vi "new Dashboard Main.vi"() -> ()   [LabVIEW 2020]
uses:
  <vilib>/Rock Robotics/Network Tables/NT Read Numeric Array.vi
panel:
  out "Camera Perf":string
  in  "Camera Settings":T1={"Frame Rate"=30, "Compression"=30, "Size"=1, "DB Camera Config"=FALSE} {"Frame Rate" scale=1.0..30.0; "Compression" scale=100.0..-1.0; "Size" items=["640x480", "320x240", "160x120"]}
  in  "TCP":refnum<k5>
  out "Robot IP":string
  in  "Dashboard Tab":enum32{"Drive", "Basic", "Custom", "Variables"}(tab)
  in  "Select Auto":string(combo)="Select Autonomous ..."
  out "NT Connection":bool
  out "MotorChart R":cluster{"Numeric":dbl, "Numeric":dbl}(graph)
  out "MotorChart L":cluster{"Numeric":dbl, "Numeric":dbl}(graph)
  out "MotorSliders R":cluster{"MotorSlide1":dbl, "MotorSlide2":dbl} {"MotorSlide2" scale=-1.0..1.0 scale format="%#_2e"; "MotorSlide1" scale=-1.0..1.0 scale format="%#_2e"}
  out "MotorSliders L":cluster{"MotorSlide1":dbl, "MotorSlide2":dbl} {"MotorSlide2" scale=-1.0..1.0 scale format="%#_2e"; "MotorSlide1" scale=-1.0..1.0 scale format="%#_2e"}
  out "JS1 Z":dbl(slide) scale=-1.0..1.0 scale format="%#_2e"
  out "JS1 Graph":cluster{"X":dbl, "Y":dbl}[](graph)
  out "JS1 Buttons":T2
  out "JS2 Z":dbl(slide) scale=-1.0..1.0 scale format="%#_2e"
  out "JS2 Graph":cluster{"X":dbl, "Y":dbl}[](graph)
  out "JS2 Buttons":T2
  out "Mode":T3(ring)=enum."Auto Disabled"
  in  "DB/String 9":string
  in  "DB/String 8":string
  in  "DB/String 7":string
  in  "DB/String 6":string
  in  "DB/String 5":string
  in  "DB/String 4":string
  in  "DB/String 3":string
  in  "DB/String 2":string
  in  "DB/String 1":string
  in  "DB/String 0":string
  in  "DB/Slider 0":dbl(slide) scale=0.0..5.0
  in  "DB/Slider 1":dbl(slide) scale=0.0..5.0
  in  "DB/Slider 2":dbl(slide) scale=0.0..5.0
  in  "DB/Slider 3":dbl(slide) scale=0.0..5.0
  out "DB/LED 3":bool
  out "DB/LED 2":bool
  out "DB/LED 1":bool
  out "DB/LED 0":bool
  in  "DB/Button 3":bool
  in  "DB/Button 2":bool
  in  "DB/Button 1":bool
  in  "DB/Button 0":bool
  out "Tree":string(tree)
  out "Camera Image":T4(plugin-control)
  out "Background":bool
  in  "Camera Name":string(combo)="No Camera Selection"
  # "HW"
  # "Joysticks"
  # "Drive Motors"
  # "Front"
  # "Right"
  # "Left"
  # "Back"
  # "This tab is a great place for autonomous settings and robot-specific values.\nPlace controls and indicators inside this tab and match name to\nDashboard Variables on robot. You can also delete this comment."
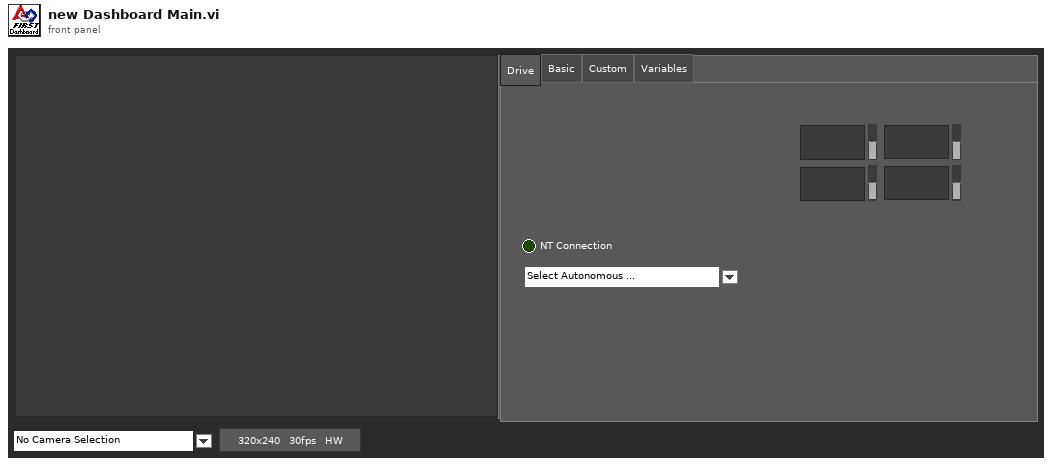
[diagram p1: front panel]
types:
  T1 = cluster{"Frame Rate":i32, "Compression":i32, "Size":u16, "DB Camera Config":bool}
  T2 = cluster{bool, bool, bool, bool, bool, bool, bool, bool, bool, bool, bool, bool}
  T3 = enum8{"Tele-Op Disabled", "Tele-Op Enabled", "Auto Disabled", "Auto Enabled", "Test Disabled", "Test Enabled", "Disconnected", "No Code", "E-Stop"}
  T4 = typedef "IMAQ Image.ctl" = refnum<image>
  T5 = cluster{"Save Path":path, "Interval (s)":dbl, "Keep":i32}
  T6 = typedef "Image Type" = u32
  T7 = cluster{"Camera Image":refnum<vi>, "Dashboard Tab":refnum<vi>, "Background":refnum<vi>, "Tree":refnum<vi>, "Camera Settings":refnum<vi>, "Camera Name":refnum<vi>, "Camera Perf":refnum<vi>}
  T8 = cluster{"Shift":bool, "Ctrl":bool, "Alt":bool, "Cmd":bool, "Opt":bool}
  T9 = cluster{"Error Strings":string, "Disable Counts":cluster{u16, u16}, "Rail Faults":cluster{u16, u16, u16}, "Robot IP":string, "DB Mode":u8, "Event Info":cluster{"Name":string, "Type":u8, "Number":u16, "Replay":u8}}
  T10 = cluster{"Storage":cluster{"Disk Free":u64, "RAM Block":u32, "RAM free":u32}, "CPU Utilization":cluster{"CPU % ISR":sgl, "CPU % Time Crit":sgl, "CPU % Timed Str":sgl, "CPU % High":sgl, "CPU % Above":sgl, "CPU % Normal":sgl, "CPU % Low":sgl}, "CAN":cluster{"% Bus Utilization":sgl, "Bus Off Cnt":u32, "TX_FIFO Full Cnt":u32, "Receive Error Cnt":u8, "Transmit Error Cnt":u8}, "HID":cluster{"HID Outputs":u32, "Rumble Low":u16, "Rumble High":u16}[]}
  T11 = cluster{"Status bits":cluster{"Test Mode":bool, "Autonomous":bool, "Enabled":bool, "Code Start":bool, "Brownout":bool, "Reserved 2":bool, "Reserved 3":bool, "E-Stop":bool}, "Code Trace":cluster{"Disabled":bool, "TeleOp":bool, "Auto":bool, "Test":bool}, "Controller Type":enum16{"unknown", "cRIO", "roboRio"}, "Code?":enum16{"unknown", "noCode", "code"}, "Battery V":dbl}
  T12 = cluster{"Control Bits":cluster{"TestMode":bool, "Autonomous":bool, "Enabled":bool, "FMS Present":bool, bool, bool, bool, "E-Stop":bool}, "Team Station ":u8, "Countdown":sgl, "Joystick Values":cluster{"Axes":dbl[], "Buttons":bool[], "POVs":i16[]}[]}
  T13 = cluster{"Axes":dbl[], "Buttons":bool[], "POVs":i16[]}[]
  T14 = cluster{"Axes":dbl[], "Buttons":bool[], "POVs":i16[]}
  T15 = cluster{"Buttons[0]":bool, "Buttons[1]":bool, "Buttons[2]":bool, "Buttons[3]":bool, "Buttons[4]":bool, "Buttons[5]":bool, "Buttons[6]":bool, "Buttons[7]":bool, "Buttons[8]":bool, "Buttons[9]":bool, "Buttons[10]":bool, "Buttons[11]":bool}
  T16 = cluster{"Camera Name":string, "Camera File Name":string, "Saved DB Images Info":cluster{"Save Path":path, "Interval (s)":dbl, "Keep":i32}}
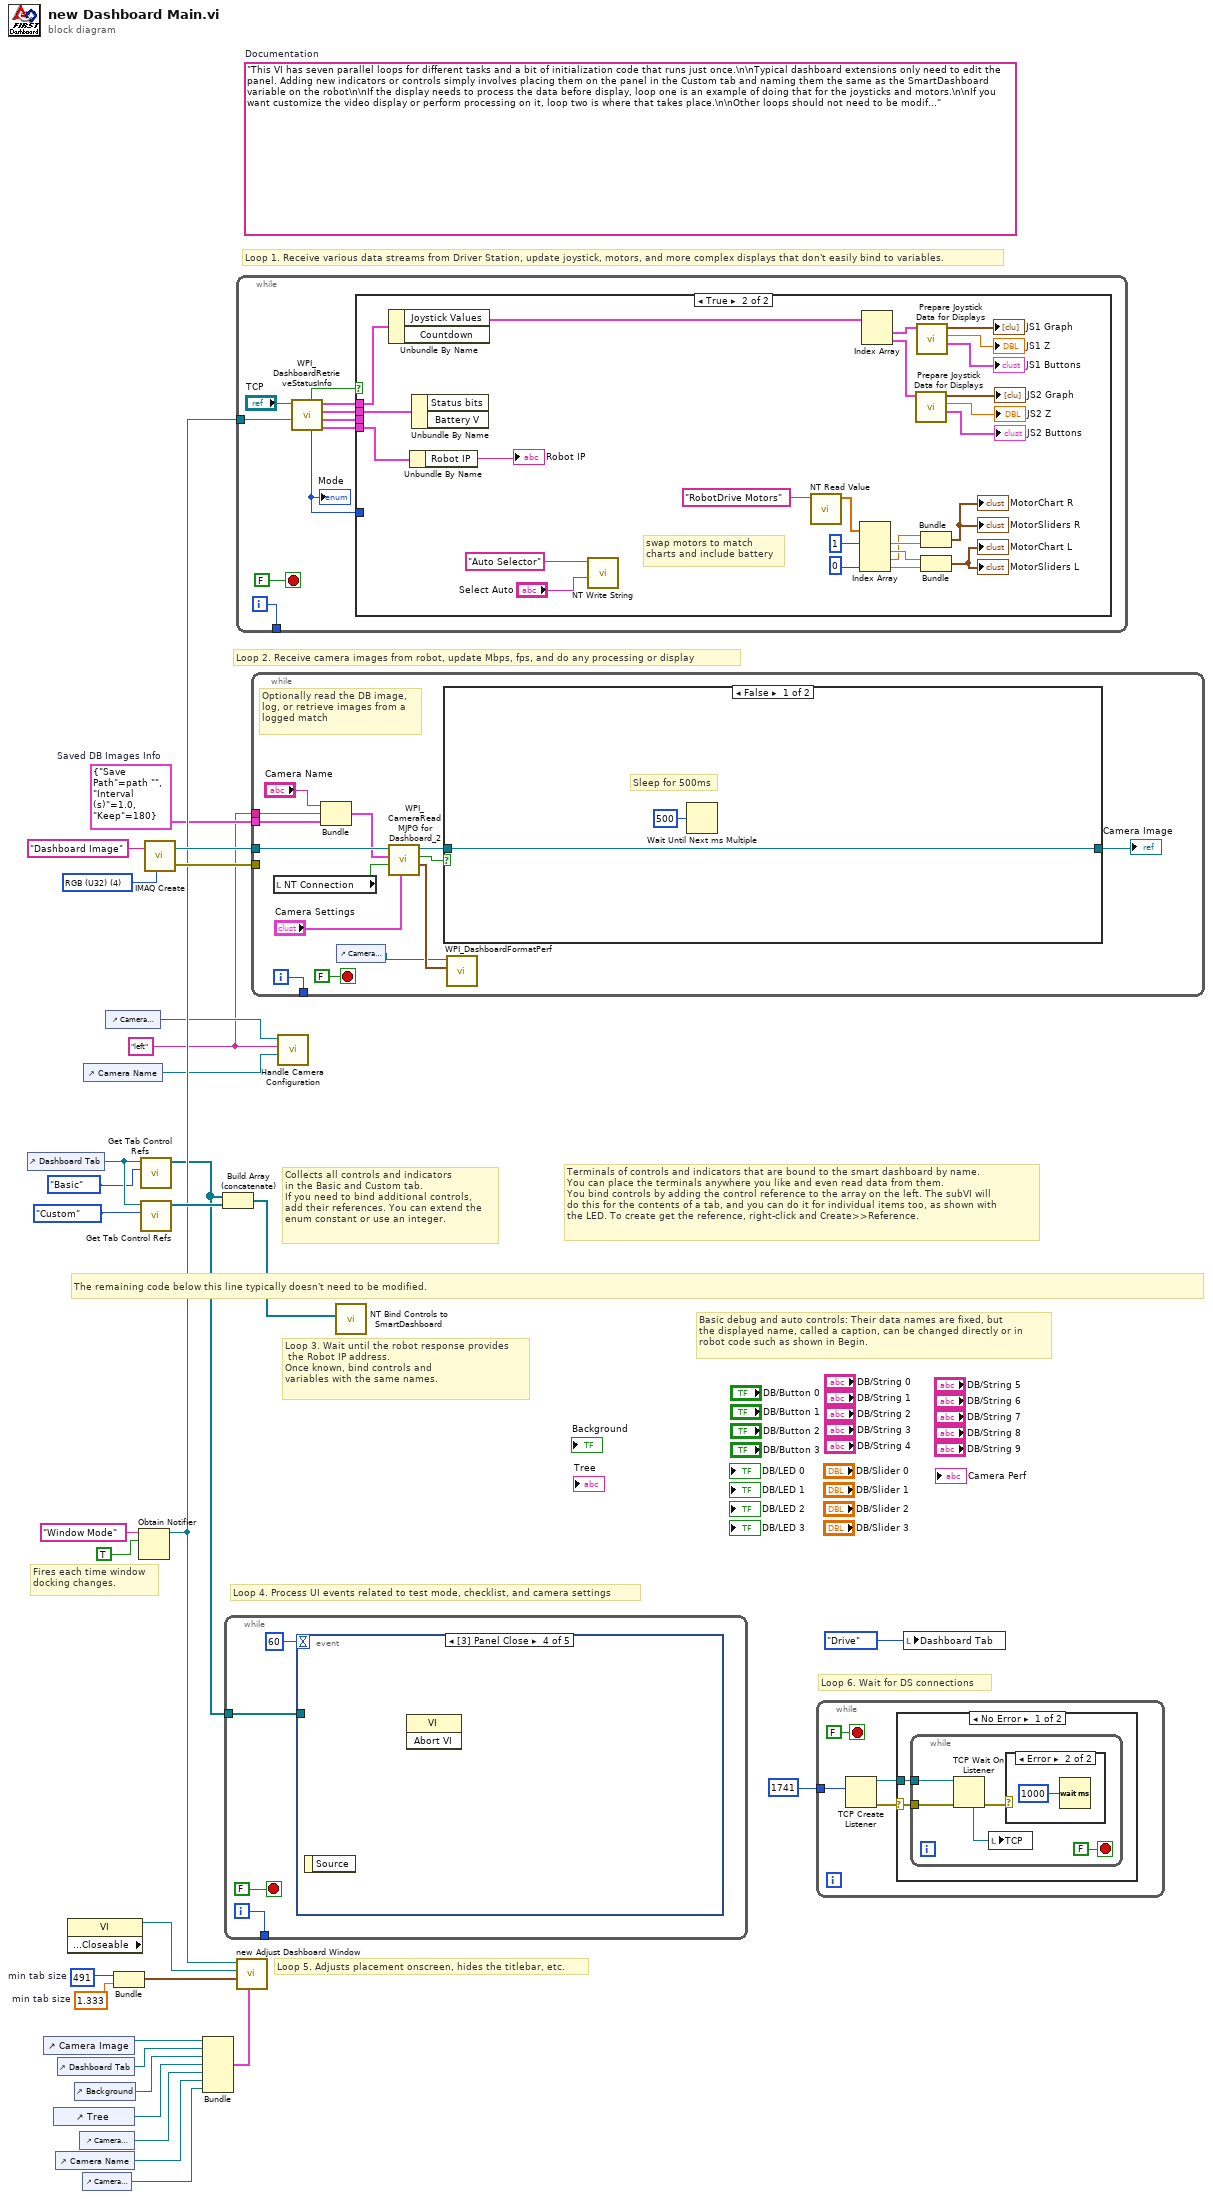
[diagram p0: block diagram]
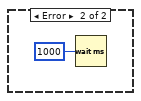
[diagram p3: hidden frame]
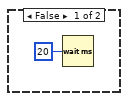
[diagram p4: hidden frame]
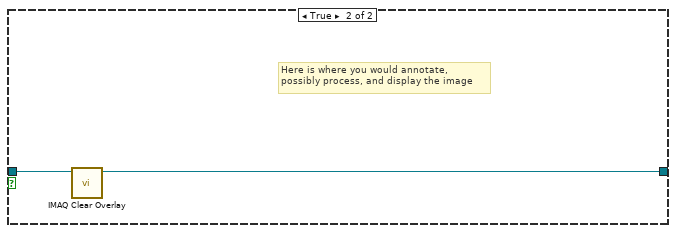
[diagram p5: hidden frame]
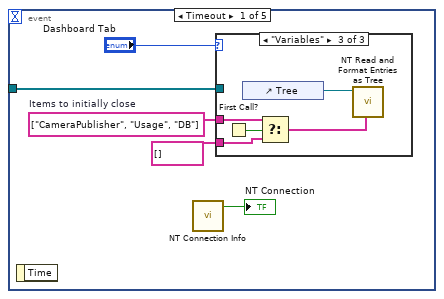
[diagram p6: hidden frame]
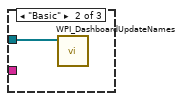
[diagram p8: hidden frame]
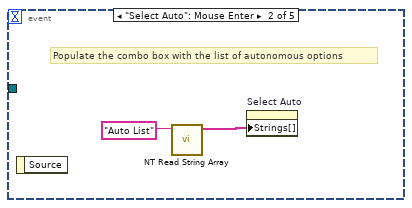
[diagram p9: hidden frame]
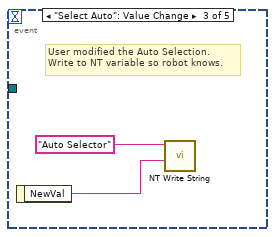
[diagram p10: hidden frame]
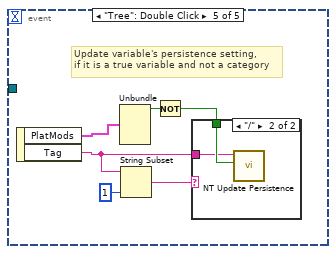
[diagram p11: hidden frame]
diagram:
  w2 = "left" ("Camera File Name")
  w3 = T5 {"Save Path"=path "", "Interval (s)"=1.0, "Keep"=180}  # Saved DB Images Info
  w19 = 491  # min tab size
  w18 = 1.333  # min tab size
  (unwired) "This VI has seven parallel loops for different tasks and a bit of initialization code that runs just once.\n\nTypical dashboard extensions only need to edit the panel. Adding new indicators or controls simply involves placing them on the panel in the Custom tab and naming them the same as the SmartDashboard variable on the robot\n\nIf the display needs to process the data before display, loop one is an example of doing that for the joysticks and motors.\n\nIf you want customize the video display or perform processing on it, loop two is where that takes place.\n\nOther loops should not need to be modified. They are pretty standard, and document the task they perform."  # Documentation
  w31 = T6 4 items=["Grayscale (U8)", "Grayscale (I16)", "Grayscale (SGL)", "Complex (CSG)", "RGB (U32)", "HSL (U32)", "RGB (U64)"] ("Image Type")
  # "Loop 6. Wait for DS connections"
  # "Basic debug and auto controls: Their data names are fixed, but\nthe displayed name, called a caption, can be changed directly or in\nrobot code such as shown in Begin."
  # "Fires each time window\ndocking changes."
  # "Collects all controls and indicators\nin the Basic and Custom tab.\nIf you need to bind additional controls,\nadd their references. You can extend the\nenum constant or use an integer."
  # "The remaining code below this line typically doesn't need to be modified."
  # "Loop 4. Process UI events related to test mode, checklist, and camera settings"
  # "Terminals of controls and indicators that are bound to the smart dashboard by name.\nYou can place the terminals anywhere you like and even read data from them.\nYou bind controls by adding the control reference to the array on the left. The subVI will\ndo this for the contents of a tab, and you can do it for individual items too, as shown with\nthe LED. To create get the reference, right-click and Create>>Reference."
  # "Loop 3. Wait until the robot response provides\n the Robot IP address.\nOnce known, bind controls and\nvariables with the same names."
  # "Loop 5. Adjusts placement onscreen, hides the titlebar, etc."
  # "Loop 1. Receive various data streams from Driver Station, update joystick, motors, and more complex displays that don't easily bind to variables."
  # "Loop 2. Receive camera images from robot, update Mbps, fps, and do any processing or display"
  n1 = control-ref of="Dashboard Tab"() -> (w24:refnum<vi>)
  n2 = control-ref of="Camera Image"() -> (w21:refnum<vi>)
  n3 = control-ref of="Tree"() -> (w9:refnum<vi>)
  n4 = control-ref of="Camera Name"() -> (w7:refnum<vi>)
  n5 = control-ref of="Dashboard Tab"() -> (w20:refnum<vi>)
  n6 = property class="VI" props=["Front Panel.Closeable"]() -> (reference out=w25:refnum<vi>)  [unwired: 2 in, 2 out]
  n7 = control-ref of="Background"() -> (w16:refnum<vi>)
  n8 = control-ref of="Camera Settings"() -> (w8:refnum<vi>)
  n9 = control-ref of="Camera Perf"() -> (w6:refnum<vi>)
  n10 = control-ref of="Camera Name"() -> (w11:refnum<vi>)
  n11 = control-ref of="Camera Settings"() -> (w12:refnum<vi>)
  n12 = Bundle("min tab size"=w19, "min tab size"=w18) -> (w17:cluster{"min tab size":i32, "min tab size":dbl})  [unwired: 1 in]
  n13 = Obtain Notifier(name (unnamed)="Window Mode", notification data type=TRUE) -> (notifier out=w14:refnum<notifier>)  [unwired: 2 in, 2 out]
  n14 = call <vilib>:"Get Tab Control Refs.vi"("Page Index"=enum32{"Drive", "Basic", "Custom", "Variables"}."Basic" ("Dashboard Tab"), "TabControl in"=w24) -> ("ControlsOnPage"=w10:refnum<vi>[])  [unwired: 9 in]
  n15 = call <vilib>:"Get Tab Control Refs.vi"("Page Index"=enum32{"Drive", "Basic", "Custom", "Variables"}."Custom" ("Dashboard Tab"), "TabControl in"=w24) -> ("ControlsOnPage"=w23:refnum<vi>[])  [unwired: 9 in]
  n16 = call "IMAQ Create"("Image Name"="Dashboard Image", "Image Type"=w31) -> ("New Image"=w29:T4, "error out"=w28:errorcluster)  [unwired: 2 in, 1 out]
  n17 = Bundle("Camera Image"=w21, "Dashboard Tab"=w20, "Background"=w16, "Tree"=w9, "Camera Settings"=w8, "Camera Name"=w7, "Camera Perf"=w6) -> (w15:T7)  [unwired: 1 in]
  n18 = Build Array (concatenate)(w10, w23) -> (w22:refnum<vi>[])
  n19 = while {
    tunnel: [w33] -> _
    tunnel: w10 -> [w32]
    i -> [w33]
    stop <- FALSE stop-if-true
    n20 = event shown="[3] Panel Close" {
      selector: _ -> [_ _ _ _ _]
      dyn-events: _ -> [_ _ _ _ _]
      timeout: u32 60 ("milliseconds to wait") -> [_ _ _ _ _]
      tunnel: w32 -> [w39 _ _ _ _]
      event Timeout {
        w38 = string[] ["CameraPublisher", "Usage", "DB"]  # Items to initially close
        n21 = event-data() -> ()  [unwired: 1 in, 1 out]
        n22 = call <vilib>:"NT Connection Info.vi"() -> ("Connected"=→"NT Connection":bool)  [unwired: 11 in]
        n23 = case shown="\"Variables\"" "Dashboard Tab" {
          tunnel: w39 -> [_ w41 _]
          tunnel: w38 -> [_ _ w44]
          tunnel: string[] [] -> [_ _ w43]
          frame "Custom", Default {
          }
          frame "Basic" {
            n24 = call <vilib>:"WPI_DashboardUpdateNames.vi"("Controls on Tab"=w41) -> ()  [unwired: 11 in]
          }
          frame "Variables" {
            n25 = First Call?() -> (First Call?: T/F=w45:bool)
            n26 = control-ref of="Tree"() -> (w46:refnum<vi>)
            n27 = Select(t=w44, s=w45, f=w43) -> (s? t:f=w42:string[])
            n28 = call <vilib>:"NT Read and Format Entries as Tree.vi"("Tags to  Close"=w42, "Tree Refnum"=w46) -> ()  [unwired: 8 in, 2 out]
          }
        }
      }
      event "Select Auto": Mouse Enter {
        # "Populate the combo box with the list of autonomous options"
        n29 = event-data() -> ()  [unwired: 1 in, 1 out]
        n30 = call <vilib>:"NT Read String Array.vi"("name"="Auto List" ("Name")) -> ("value"=w47:string[])  [unwired: 8 in, 2 out]
        n31 = property on="Select Auto" class="CmbBox"("Strings[]"=w47) -> ()  [unwired: 2 in, 2 out]
      }
      event "Select Auto": Value Change {
        # "User modified the Auto Selection.\nWrite to NT variable so robot knows."
        n32 = event-data() -> ("NewVal"=w49:string)  [unwired: 1 in]
        n33 = call <vilib>:"NT Write String.vi"("value"=w49, "name"="Auto Selector" ("Name")) -> ()  [unwired: 9 in, 1 out]
      }
      event Panel Close {
        n34 = event-data() -> ()  [unwired: 1 in, 1 out]
        n35 = invoke class="VI" method="Abort VI"() -> ()  [unwired: 3 in, 3 out]
      }
      event "Tree": Double Click {
        # "Update variable's persistence setting,\nif it is a true variable and not a category"
        n36 = event-data() -> ("PlatMods"=w52:T8, "Tag"=w51:string)  [unwired: 1 in]
        n37 = Unbundle(w52) -> ("Shift"=w56:bool)  [unwired: 4 out]
        n38 = String Subset(string=w51, length (rest)=1 ("length (rest)")) -> (substring=w53:string)  [unwired: 1 in]
        n39 = Not(x=w56) -> (.not. x?=w55:bool)
        n40 = case shown="\"/\"" w53 {
          tunnel: w55 -> [_ w58]
          tunnel: w51 -> [_ w57]
          frame Default {
          }
          frame "/" {
            n41 = call <vilib>:"NT Update Persistence.vi"("Persistence"=w58, "Name"=w57) -> ()  [unwired: 9 in, 1 out]
          }
        }
      }
    }
  }
  n42 = while {
    tunnel: [w67] -> _
    tunnel: w14 -> [w59]
    i -> [w67]
    stop <- FALSE stop-if-true
    n43 = call <vilib>:"WPI_DashboardRetrieveStatusInfo.vi"("Window Mode Notifier"=w59, "TCP Cnx"="TCP") -> ("Power and Errors"=w62:T9, "Robot Metrics"=w65:T10, "Status Info"=w66:T11, "Control Info"=w63:T12, "Robot Mode"=w61:T3, "Process?"=w64:bool)  [unwired: 4 in]
    "Mode" <- w61
    n44 = case shown="True" w64 {
      tunnel: w66 -> [_ w94]
      tunnel: w65 -> [_ _]
      tunnel: w63 -> [_ w93]
      tunnel: w62 -> [_ w92]
      tunnel: w61 -> [_ _]
      frame False {
        n45 = Wait (ms)(milliseconds to wait=u32 20) -> ()  [unwired: 1 out]
      }
      frame True {
        # "swap motors to match\ncharts and include battery"
        n46 = Unbundle By Name(w93) -> ("Joystick Values"=w83:T13)  [unwired: 1 out]
        n47 = Unbundle By Name(w92) -> ("Robot IP"=→"Robot IP":string)
        n48 = Unbundle By Name(w94) -> ()  [unwired: 2 out]
        n49 = call <vilib>:"NT Write String.vi"("value"="Select Auto", "name"="Auto Selector" ("Name")) -> ()  [unwired: 9 in, 1 out]
        n50 = call-poly <vilib>:"NT Read Value.vi"("name"="RobotDrive Motors" ("Name")) -> ("value"=w73:dbl[])  [unwired: 8 in, 2 out]
        n51 = Index Array(array=w73, index #1=1, index #4=0) -> (element #1=w87:dbl, element #2=w88:dbl, element #3=w86:dbl, element #4=w91:dbl)  [unwired: 2 in]
        n52 = Index Array(array=w83) -> (element #1=w82:T14, element #2=w78:T14)  [unwired: 2 in]
        n53 = call "Prepare Joystick Data for Displays.vi"("Joystick Values"=w78) -> ("Buttons"=→"JS2 Buttons":T15, "Z Axis"=→"JS2 Z":dbl, "Cartesian Data"=→"JS2 Graph":cluster{"X axis":dbl, "X axis":dbl}[])  [unwired: 8 in]
        n54 = call "Prepare Joystick Data for Displays.vi"("Joystick Values"=w82) -> ("Buttons"=→"JS1 Buttons":T15, "Z Axis"=→"JS1 Z":dbl, "Cartesian Data"=→"JS1 Graph":cluster{"X axis":dbl, "X axis":dbl}[])  [unwired: 8 in]
        n55 = Bundle("Numeric"=w86, "Numeric"=w87) -> (→"MotorChart R" →"MotorSliders R":cluster{"Numeric":dbl, "Numeric":dbl})  [unwired: 1 in]
        n56 = Bundle("Numeric"=w88, "Numeric"=w91) -> (→"MotorChart L" →"MotorSliders L":cluster{"Numeric":dbl, "Numeric":dbl})  [unwired: 1 in]
      }
    }
  }
  n57 = call "new Adjust Dashboard Window.vi"("Sizing Refnums"=w15, "Size Constraints"=w17, "VI"=w25, "WIn Mode"=w14) -> ()  [unwired: 8 in]
  n58 = while {
    tunnel: w29 -> [w106]
    tunnel: w28 -> [_]
    tunnel: [w107] -> _
    tunnel: w3 -> [w100]
    tunnel: w2 -> [w97]
    i -> [w107]
    stop <- FALSE stop-if-true
    # "Optionally read the DB image,\nlog, or retrieve images from a\nlogged match"
    n59 = local read "NT Connection"() -> (w101:bool)
    n60 = Bundle("Camera Name"="Camera Name", "Camera File Name"=w97, "Saved DB Images Info"=w100) -> (w99:T16)  [unwired: 1 in]
    n61 = control-ref of="Camera Perf"() -> (w95:refnum<vi>)
    n62 = call <vilib>:"WPI_CameraRead MJPG for Dashboard_2.vi"("Camera Settings"="Camera Settings", "NT Connection"=w101, "Capture Info"=w99, "Image in"=w106) -> ("perf info"=w96:cluster{"Bandwidth (Mbps)":dbl, "fps":dbl}, "Active"=w104:bool, "Image\\ out"=w105:T4)  [unwired: 5 in]
    n63 = case shown="False" w104 {
      tunnel: w105 -> [w109 w112]
      tunnel: [w109 w111] -> w102
      frame False {
        # "Sleep for 500ms"
        n64 = Wait Until Next ms Multiple(millisecond multiple=u32 500) -> ()  [unwired: 1 out]
      }
      frame True {
        # "Here is where you would annotate,\npossibly process, and display the image"
        n65 = call "IMAQ Clear Overlay"("Image"=w112) -> ("Image Out"=w111:T4)  [unwired: 2 in, 8 out]
      }
    }
    "Camera Image" <- w102
    n66 = call <vilib>:"WPI_DashboardFormatPerf.vi"("Performance"=w96, "String in"=w95) -> ()  [unwired: 10 in]
  }
  n67 = call "Handle Camera Configuration.vi"("CameraNameRef"=w11, "Display Name"=w2, "ClusterRef"=w12) -> ()  [unwired: 9 in]
  n68 = call <vilib>:"NT Bind Controls to SmartDashboard.vi"("Bound Control Refs"=w22) -> ()  [unwired: 11 in]
  n69 = while {
    tunnel: u16 1741 ("timeout ms (25000)") -> [w114]
    stop <- FALSE stop-if-true
    n70 = TCP Create Listener(10:w114) -> (0:w113:errorcluster, 3:w115:refnum<k5>)  [unwired: 4 in, 1 out]
    n71 = case shown="No Error" w113 {
      selector: w113 -> [w117 _]
      tunnel: w115 -> [w118 _]
      frame No Error {
        n72 = while {
          tunnel: w118 -> [w121]
          tunnel: w117 -> [w120]
          stop <- FALSE stop-if-true
          n73 = TCP Wait On Listener(8:w120, 11:w121) -> (0:w122:errorcluster, 4:w123:refnum<k5>)  [unwired: 2 in, 3 out]
          n74 = local write "TCP"(w123) -> ()
          n75 = case shown="Error" w122 {
            frame No Error {
            }
            frame Error {
              n76 = Wait (ms)(milliseconds to wait=u32 1000) -> ()  [unwired: 1 out]
            }
          }
        }
      }
      frame Error {
        n77 = Wait (ms)(milliseconds to wait=u32 1000) -> ()  [unwired: 1 out]
      }
    }
  }
  n78 = local write "Dashboard Tab"(enum32{"Drive", "Basic", "Custom", "Variables"}."Drive" ("Dashboard Tab")) -> ()
